vi "subVIerror.vi"(8 "first error":errorcluster) -> (0 "second \nerror":errorcluster, 1 "x*y":dbl)   [LabVIEW 2015]
doc: "This VI will create a random number between 1 and 5 and it'll print an error if there exists any"
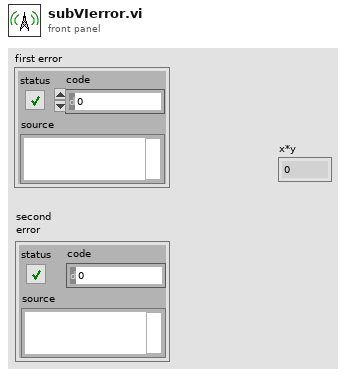
[diagram p1: front panel]
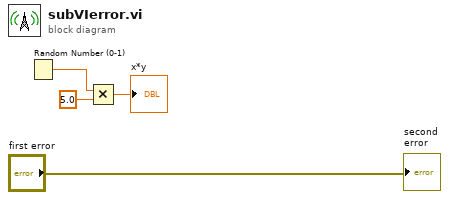
[diagram p0: block diagram]
diagram:
  n1 = Random Number (0-1)() -> (number: 0 to 1=w2:dbl)
  n2 = Multiply(x=w2, y=5.0) -> (x*y=→"x*y":dbl)
  "second \nerror" <- "first error"
